vi "VisionExecute.v.vi"(8 "error in (no error)":errorcluster) -> (0 "error out":errorcluster)   [LabVIEW 2025]
uses:
  <vilib>/Rock Robotics/WPI/ThirdParty/JAS_Junk/TrajLib/Trajectory_Library.lvlib
  <vilib>/Rock Robotics/WPI/ThirdParty/PhotonVisionLib/PhotonVisionLib.lvlib
  <vilib>/Rock Robotics/WPI/ThirdParty/PhotonVisionLib/Enum/PhotonPoseStrategy_ENUM.ctl
  VisionGlobal.vi
  <vilib>/Rock Robotics/WPI/ThirdParty/JAS_Junk/TrajLib/TypeDef/TRANSLATION2D.ctl
  <vilib>/Rock Robotics/WPI/ThirdParty/JAS_Junk/TrajLib/TypeDef/ROTATION2D.ctl
  <vilib>/Rock Robotics/WPI/ThirdParty/JAS_Junk/TrajLib/TypeDef/POSE2D.ctl
  VisionNetworkingGlobal.vi
  <vilib>/Rock Robotics/Network Tables/NT Write Number.vi
  <vilib>/Rock Robotics/WPI/ThirdParty/JAS_Junk/TrajLib/VI/AprilTagFieldLayout_New2026AndyMark.vi
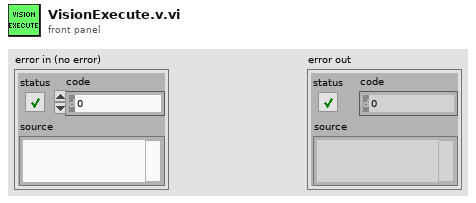
[diagram p1: front panel]
types:
  T1 = typedef "PhotonVisionLib.lvlib/PhotonPoseStrategy_ENUM.ctl" = enum16{"LOWEST_AMBIGUITY", "CLOSEST_TO_CAMERA_HEIGHT", "CLOSEST_TO_REFERENCE_POSE", "CLOSEST_TO_LAST_POSE", "AVERAGE_BEST_TARGETS", "MULTI_TAG_PNP_ON_COPROCESSOR", "MULTI_TAG_PNP_ON_RIO", "PNP_DISTANCE_TRIG_SOLVE", "CONSTRAINED_SOLVEPNP"}
  T2 = typedef "Trajectory_Library.lvlib/TRANSLATION3D.ctl" = cluster{"X":dbl, "Y":dbl, "Z":dbl}
  T3 = typedef "Trajectory_Library.lvlib/ROTATION3D.ctl" = cluster{"Q_quaternion":T4}
  T4 = typedef "Trajectory_Library.lvlib/QUATERNION.ctl" = cluster{"R":dbl, "V":dbl[]}
  T5 = typedef "Trajectory_Library.lvlib/TRANSFORM3D.ctl" = cluster{"TRANSLATION3D":T2, "ROTATION3D":T3, "XF":bool}
  T6 = typedef "PhotonVisionLib.lvlib/PhotonPipelineResultType.ctl" = cluster{"Targets":T7[], "PhotonMultiTargetPNPResult":T9, "PhotonPipelineMetadata":T11}
  T7 = typedef "PhotonVisionLib.lvlib/PhotonTrackedTargetType.ctl" = cluster{"Yaw":dbl, "Pitch":dbl, "Area":dbl, "Skew":dbl, "MinAreaRectCorners":T8[], "BestCameraToTarget":T5, "FiducialId":i32, "AltCameraToTarget":T5, "PoseAmbiguity":dbl, "DetectedCorners":T8[], "ObjDetectId":i32, "ObjDetectConf":sgl}
  T8 = typedef "PhotonVisionLib.lvlib/TargetCornerType.ctl" = cluster{"X":dbl, "Y":dbl}
  T9 = typedef "PhotonVisionLib.lvlib/PhotonMultiTargetPNPResultType.ctl" = cluster{"PhotonPNPResult":T10, "FiducialIDsUsed":i16[]}
  T10 = typedef "PhotonVisionLib.lvlib/PhotonPNPResultType.ctl" = cluster{"IsPresent":bool, "bestReprojErr":dbl, "altReprojErr":dbl, "ambiguity":dbl, "Best":T5, "Alt":T5}
  T11 = typedef "PhotonVisionLib.lvlib/PhotonPipelineMetadataType.ctl" = cluster{"CaptureTimestampMicros":i64, "PublishTimestampMicros":i64, "SequenceID":i64, "TimeSinceLastPong":i64}
  T12 = typedef "Trajectory_Library.lvlib/AprilTagFieldLayout.ctl" = cluster{"AprilTagMap":map{i32, T13}, "FieldLength":dbl, "FieldWidth":dbl, "OriginPosition ":T15, "OriginPose3d":T14}
  T13 = typedef "Trajectory_Library.lvlib/AprilTag.ctl" = cluster{"ID":i32, "POSE3D":T14}
  T14 = typedef "Trajectory_Library.lvlib/POSE3D.ctl" = cluster{"Translation3d":T2, "Rotation3d":T3}
  T15 = typedef "Trajectory_Library.lvlib/AprilTagFieldLayoutOrignPosition_ENUM.ctl" = enum16{"kBlueAllianceWallRightSide,", "kRedAllianceWallRightSide,"}
  T16 = typedef "Trajectory_Library.lvlib/POSE2D.ctl" = cluster{"TRANSLATION":T17, "ROTATION":T18}
  T17 = typedef "Trajectory_Library.lvlib/TRANSLATION2D.ctl" = cluster{"X":dbl, "Y":dbl}
  T18 = typedef "Trajectory_Library.lvlib/ROTATION2D.ctl" = cluster{"VALUE":dbl, "COS":dbl, "SIN":dbl}
  T19 = typedef "PhotonVisionLib.lvlib/PhotonPoseEstimator_Configuration.ctl" = cluster{"Primary Strategy":T1, "Camera":string, "Initial Pose":T14, "HighestAmbiguity":dbl, "RobotToCamera":T5, "FallBack Strategy":T1, "BaseNTName":string}
  T20 = typedef "Trajectory_Library.lvlib/SWERVE_DRIVE_KINEMATICS.ctl" = cluster{"NumModules":i32, "InverseKinematics":T21, "ForwardKinematics":T21, "Modules":T17[], "PrevCoR":T17, "SavedModuleStates":T22[]}
  T21 = typedef "NI_Matrix.lvlib/RealMatrix.ctl" = dbl[][]
  T22 = typedef "Trajectory_Library.lvlib/SWERVE_DRIVE_MODULE_STATE.ctl" = cluster{"Speed":dbl, "Angle":T18}
  T23 = typedef "Trajectory_Library.lvlib/SWERVE_DRIVE_MODULE_POSITION.ctl" = cluster{"Distance":dbl, "Angle":T18, "P":bool}
  T24 = typedef "Trajectory_Library.lvlib/SWERVE_DRIVE_POSE_EST2_CONFIG.ctl" = cluster{"Wheel_Locations M":T17[], "Odom X std dev M":dbl, "Odom Y std dev M":dbl, "Odom Heading std dev Rad":dbl, "Vision X std dev M":dbl, "Vision Y std dev M":dbl, "Vision Heading std dev Rad":dbl}
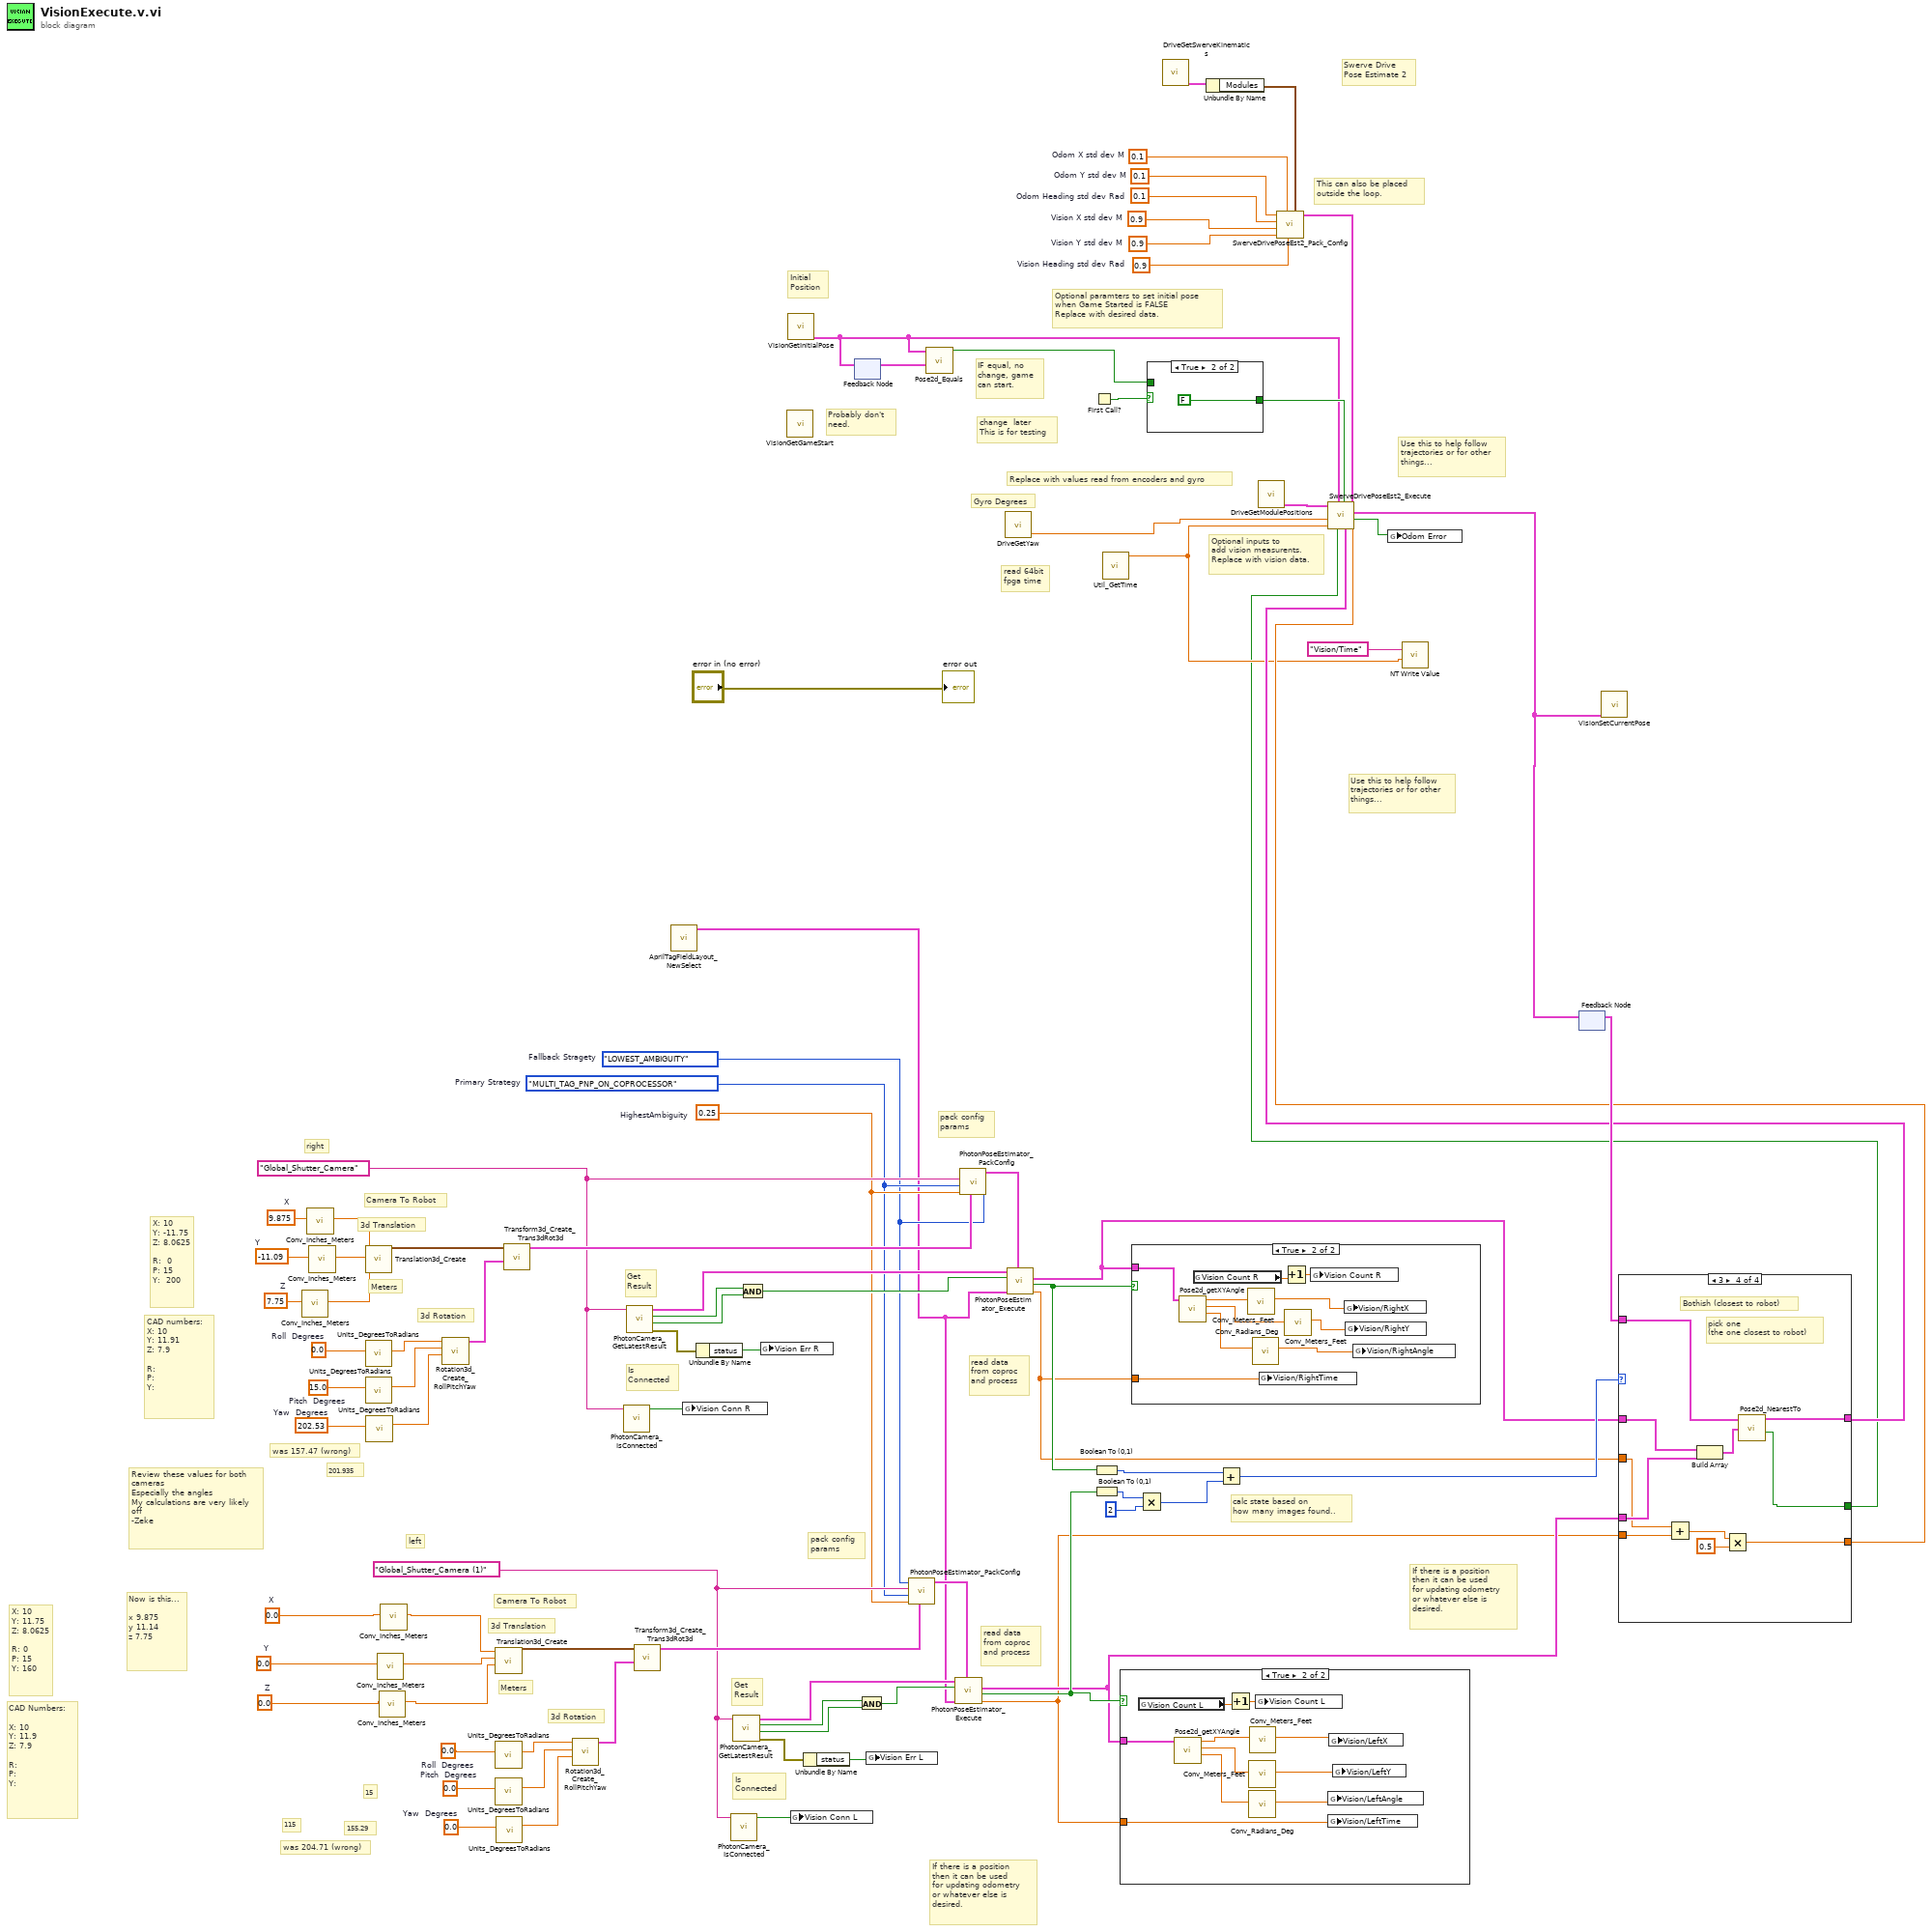
[diagram p0: block diagram]
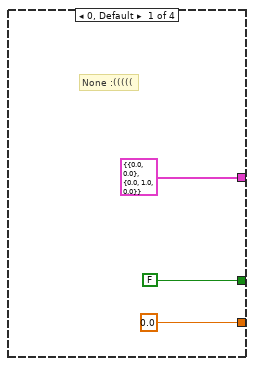
[diagram p3: hidden frame]
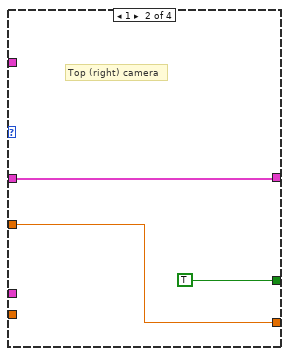
[diagram p4: hidden frame]
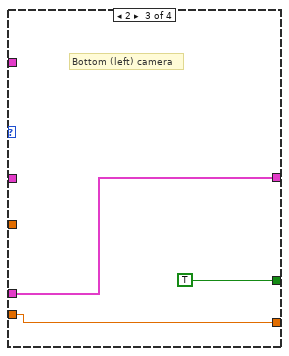
[diagram p5: hidden frame]
diagram:
  w15 = PhotonPoseStrategy_ENUM."LOWEST_AMBIGUITY"  # Fallback Stragety
  w25 = 0.1  # Odom Y std dev M
  w26 = 0.1  # Odom Heading std dev Rad
  w27 = 0.9  # Vision X std dev M
  w28 = 0.9  # Vision Y std dev M
  w29 = 0.1  # Odom X std dev M
  w30 = 0.9  # Vision Heading std dev Rad
  w63 = 0.0  # Roll  Degrees
  w62 = 0.0  # Pitch  Degrees
  w61 = 0.0  # Yaw  Degrees
  w48 = 0.0  # Z
  w52 = 0.0  # X
  w50 = 0.0  # Y
  w57 = "Global_Shutter_Camera (1)" ("CameraName")
  w81 = 0.0  # Roll  Degrees
  w80 = 15.0  # Pitch  Degrees
  w79 = 202.53  # Yaw  Degrees
  w42 = 7.75  # Z
  w46 = 9.875  # X
  w44 = -11.09  # Y
  w40 = 0.25  # HighestAmbiguity
  w39 = PhotonPoseStrategy_ENUM."MULTI_TAG_PNP_ON_COPROCESSOR"  # Primary Strategy
  w75 = "Global_Shutter_Camera" ("CameraName")
  # "calc state based on\nhow many images found.."
  # "read data\nfrom coproc\nand process"
  # "read data\nfrom coproc\nand process"
  # "pack config\nparams"
  # "pack config\nparams"
  # "15"
  # "155.29"
  # "Now is this...\n\nx 9.875\ny 11.14\nz 7.75"
  # "115"
  # "was 157.47 (wrong)"
  # "was 204.71 (wrong)"
  # "CAD Numbers:\n\nX: 10 \nY: 11.9\nZ: 7.9\n\nR:\nP:\nY:"
  # "CAD numbers:\nX: 10\nY: 11.91\nZ: 7.9\n\nR:\nP:\nY:"
  # "X: 10\nY: 11.75\nZ: 8.0625\n\nR: 0\nP: 15\nY: 160"
  # "X: 10 \nY: -11.75\nZ: 8.0625\n\nR:  0\nP: 15\nY:  200"
  # "Probably don't\nneed."
  # "IF equal, no \nchange, game\ncan start."
  # "Initial\nPosition"
  # "201.935"
  # "change  later\nThis is for testing"
  # "Review these values for both cameras\nEspecially the angles\nMy calculations are very likely off\n-Zeke"
  # "Optional inputs to\nadd vision measurents.\nReplace with vision data."
  # "Replace with values read from encoders and gyro"
  # "Optional paramters to set initial pose\nwhen Game Started is FALSE\nReplace with desired data."
  # "read 64bit\nfpga time"
  # "This can also be placed \noutside the loop."
  # "Use this to help follow\ntrajectories or for other\nthings..."
  # "Swerve Drive \nPose Estimate 2"
  # "Use this to help follow\ntrajectories or for other\nthings..."
  # "right"
  # "left"
  # "If there is a position\nthen it can be used\nfor updating odometry\nor whatever else is \ndesired."
  # "Meters"
  # "Camera To Robot"
  # "3d Rotation"
  # "3d Translation"
  # "Is\nConnected"
  # "Get\nResult"
  # "If there is a position\nthen it can be used\nfor updating odometry\nor whatever else is \ndesired."
  # "Meters"
  # "Camera To Robot"
  # "3d Rotation"
  # "3d Translation"
  # "Is\nConnected"
  # "Get\nResult"
  # "Gyro Degrees"
  n1 = call <vilib>:"Conv_Inches_Meters.vi"("INCH"=w42) -> ("Meters"=w41:dbl)  [unwired: 10 in]
  n2 = call <vilib>:"Conv_Inches_Meters.vi"("INCH"=w46) -> ("Meters"=w45:dbl)  [unwired: 10 in]
  n3 = call <vilib>:"Conv_Inches_Meters.vi"("INCH"=w44) -> ("Meters"=w43:dbl)  [unwired: 10 in]
  n4 = call <vilib>:"Translation3d_Create.vi"("Z"=w41, "Y"=w43, "X"=w45) -> ("TRANSLATION3D"=w82:T2)  [unwired: 8 in]
  n5 = call <vilib>:"Units_DegreesToRadians.vi"("Degrees"=w81) -> ("Radians"=w78:dbl)  [unwired: 10 in]
  n6 = call <vilib>:"Units_DegreesToRadians.vi"("Degrees"=w80) -> ("Radians"=w77:dbl)  [unwired: 10 in]
  n7 = call <vilib>:"Units_DegreesToRadians.vi"("Degrees"=w79) -> ("Radians"=w76:dbl)  [unwired: 10 in]
  n8 = call <vilib>:"Conv_Inches_Meters.vi"("INCH"=w50) -> ("Meters"=w49:dbl)  [unwired: 10 in]
  n9 = call <vilib>:"Conv_Inches_Meters.vi"("INCH"=w48) -> ("Meters"=w47:dbl)  [unwired: 10 in]
  n10 = call <vilib>:"Conv_Inches_Meters.vi"("INCH"=w52) -> ("Meters"=w51:dbl)  [unwired: 10 in]
  n11 = call <vilib>:"Rotation3d_Create_RollPitchYaw.vi"("Yaw"=w76, "Pitch"=w77, "Roll"=w78) -> ("Rotation3d"=w83:T3)  [unwired: 8 in]
  n12 = call <vilib>:"Translation3d_Create.vi"("Z"=w47, "Y"=w49, "X"=w51) -> ("TRANSLATION3D"=w64:T2)  [unwired: 8 in]
  n13 = call <vilib>:"Units_DegreesToRadians.vi"("Degrees"=w63) -> ("Radians"=w60:dbl)  [unwired: 10 in]
  n14 = call <vilib>:"Units_DegreesToRadians.vi"("Degrees"=w62) -> ("Radians"=w59:dbl)  [unwired: 10 in]
  n15 = call <vilib>:"Units_DegreesToRadians.vi"("Degrees"=w61) -> ("Radians"=w58:dbl)  [unwired: 10 in]
  n16 = call <vilib>:"Transform3d_Create_Trans3dRot3d.vi"("Rotation3d"=w83, "Translation3d"=w82) -> ("Transform3d"=w84:T5)  [unwired: 9 in]
  n17 = call <vilib>:"Rotation3d_Create_RollPitchYaw.vi"("Yaw"=w58, "Pitch"=w59, "Roll"=w60) -> ("Rotation3d"=w65:T3)  [unwired: 8 in]
  n18 = call <vilib>:"PhotonCamera_IsConnected.vi"("CameraName"=w75) -> ("IsConnected"=w73:bool)  [unwired: 9 in, 1 out]
  n19 = call <vilib>:"PhotonCamera_GetLatestResult.vi"("CameraName"=w75) -> ("error out"=w72:errorcluster, "New Data"=w88:bool, "HasTargets"=w87:bool, "PipelineResult"=w85:T6)  [unwired: 6 in, 1 out]
  n20 = call <vilib>:"Transform3d_Create_Trans3dRot3d.vi"("Rotation3d"=w65, "Translation3d"=w64) -> ("Transform3d"=w66:T5)  [unwired: 9 in]
  n21 = call-poly <vilib>:"AprilTagFieldLayout_NewSelect.vi"() -> ("AprilTagFieldLayout"=w1:T12)  [unwired: 11 in]
  n22 = global write "VisionGlobal.vi" "Vision Conn R"(w73) -> ()
  n23 = Unbundle By Name(w72) -> ("status"=w71:bool)
  n24 = call <vilib>:"PhotonCamera_IsConnected.vi"("CameraName"=w57) -> ("IsConnected"=w55:bool)  [unwired: 9 in, 1 out]
  n25 = call <vilib>:"PhotonCamera_GetLatestResult.vi"("CameraName"=w57) -> ("error out"=w54:errorcluster, "New Data"=w70:bool, "HasTargets"=w69:bool, "PipelineResult"=w67:T6)  [unwired: 6 in, 1 out]
  n26 = And(x=w87, y=w88) -> (x .and. y?=w86:bool)
  n27 = global write "VisionGlobal.vi" "Vision Err R"(w71) -> ()
  n28 = call "VisionGetGameStart.vi"() -> ()  [unwired: 11 in, 1 out]
  n29 = call "VisionGetInitialPose.vi"() -> ("InitialPose"=w5:T16)  [unwired: 10 in]
  n30 = global write "VisionGlobal.vi" "Vision Conn L"(w55) -> ()
  n31 = Unbundle By Name(w54) -> ("status"=w53:bool)
  n32 = feedback-in #1(w5) -> ()
  n33 = feedback #1() -> (w4:T16)  [unwired: 1 in]
  n34 = And(x=w69, y=w70) -> (x .and. y?=w68:bool)
  n35 = global write "VisionGlobal.vi" "Vision Err L"(w53) -> ()
  n36 = call <vilib>:"PhotonPoseEstimator_PackConfig.vi"("FallBack Strategy"=w15, "RobotToCamera"=w66, "HighestAmbiguity"=w40, "PirmaryStrategy"=w39, "Camera"=w57) -> ("PoseEstimator_Configuration"=w56:T19)  [unwired: 6 in]
  n37 = call <vilib>:"Pose2d_Equals.vi"("other POSE"=w4, "in POSE"=w5) -> ("Equals"=w3:bool)  [unwired: 9 in]
  n38 = call <vilib>:"PhotonPoseEstimator_Execute.vi"("Configuration"=w56, "AprilTagFieldLayout"=w1, "PIpeline Has \nNew Results"=w68, "PipelineResult"=w67) -> ("TimeStamp_Seconds"=w10:dbl, "New Pose Found"=w37:bool, "EstimatedPose2d"=w12:T16)  [unwired: 1 in, 4 out]
  n39 = call <vilib>:"PhotonPoseEstimator_PackConfig.vi"("FallBack Strategy"=w15, "RobotToCamera"=w84, "HighestAmbiguity"=w40, "PirmaryStrategy"=w39, "Camera"=w75) -> ("PoseEstimator_Configuration"=w74:T19)  [unwired: 6 in]
  n40 = call "DriveGetYaw.vi"() -> ("Yaw"=w20:dbl)  [unwired: 11 in]
  n41 = call <vilib>:"PhotonPoseEstimator_Execute.vi"("Configuration"=w74, "AprilTagFieldLayout"=w1, "PIpeline Has \nNew Results"=w86, "PipelineResult"=w85) -> ("TimeStamp_Seconds"=w9:dbl, "New Pose Found"=w38:bool, "EstimatedPose2d"=w11:T16)  [unwired: 1 in, 4 out]
  n42 = First Call?() -> (First Call?: T/F=w13:bool)
  n43 = Boolean To (0,1)(Boolean=w38) -> (0, 1=w33:i16)
  n44 = Boolean To (0,1)(Boolean=w37) -> (0, 1=w36:i16)
  n45 = call <vilib>:"Util_GetTime.vi"() -> ("FPGA_Time_Seconds"=w7:dbl)  [unwired: 9 in, 2 out]
  n46 = case shown="True" w37 {
    tunnel: w12 -> [_ w96]
    tunnel: w10 -> [_ w95]
    frame False {
    }
    frame True {
      n47 = global read "VisionGlobal.vi" "Vision Count L"() -> (w97:dbl)
      n48 = call <vilib>:"Pose2d_getXYAngle.vi"("in POSE"=w96) -> ("Angle"=w90:dbl, "Y"=w92:dbl, "X"=w94:dbl)  [unwired: 8 in]
      n49 = Increment(x=w97) -> (x+1=w98:dbl)
      n50 = call <vilib>:"Conv_Meters_Feet.vi"("Meters"=w92) -> ("Feet"=w91:dbl)  [unwired: 10 in]
      n51 = call <vilib>:"Conv_Radians_Deg.vi"("Radians"=w90) -> ("Degrees"=w89:dbl)  [unwired: 10 in]
      n52 = call <vilib>:"Conv_Meters_Feet.vi"("Meters"=w94) -> ("Feet"=w93:dbl)  [unwired: 10 in]
      n53 = global write "VisionGlobal.vi" "Vision Count L"(w98) -> ()
      n54 = global write "VisionNetworkingGlobal.vi" "Vision/LeftAngle"(w89) -> ()
      n55 = global write "VisionNetworkingGlobal.vi" "Vision/LeftTime"(w95) -> ()
      n56 = global write "VisionNetworkingGlobal.vi" "Vision/LeftX"(w93) -> ()
      n57 = global write "VisionNetworkingGlobal.vi" "Vision/LeftY"(w91) -> ()
    }
  }
  n58 = case shown="True" w38 {
    tunnel: w11 -> [_ w106]
    tunnel: w9 -> [_ w105]
    frame False {
    }
    frame True {
      n59 = call <vilib>:"Pose2d_getXYAngle.vi"("in POSE"=w106) -> ("Angle"=w100:dbl, "Y"=w102:dbl, "X"=w104:dbl)  [unwired: 8 in]
      n60 = global read "VisionGlobal.vi" "Vision Count R"() -> (w107:dbl)
      n61 = call <vilib>:"Conv_Meters_Feet.vi"("Meters"=w104) -> ("Feet"=w103:dbl)  [unwired: 10 in]
      n62 = call <vilib>:"Conv_Radians_Deg.vi"("Radians"=w100) -> ("Degrees"=w99:dbl)  [unwired: 10 in]
      n63 = global write "VisionNetworkingGlobal.vi" "Vision/RightTime"(w105) -> ()
      n64 = Increment(x=w107) -> (x+1=w108:dbl)
      n65 = call <vilib>:"Conv_Meters_Feet.vi"("Meters"=w102) -> ("Feet"=w101:dbl)  [unwired: 10 in]
      n66 = global write "VisionGlobal.vi" "Vision Count R"(w108) -> ()
      n67 = global write "VisionNetworkingGlobal.vi" "Vision/RightX"(w103) -> ()
      n68 = global write "VisionNetworkingGlobal.vi" "Vision/RightY"(w101) -> ()
      n69 = global write "VisionNetworkingGlobal.vi" "Vision/RightAngle"(w99) -> ()
    }
  }
  n70 = Multiply(x=w36, y=i16 2) -> (x*y=w34:i16)
  n71 = case shown="True" w13 {
    tunnel: [w109 FALSE] -> w14
    tunnel: w3 -> [w109 _]
    frame False {
    }
    frame True {
    }
  }
  n72 = call "DriveGetSwerveKinematics.vi"() -> ("SWERVE_DRIVE_KINEMATICS"=w17:T20)  [unwired: 11 in]
  n73 = Unbundle By Name(w17) -> ("Modules"=w16:T17[])
  n74 = Add(x=w33, y=w34) -> (x+y=w32:i16)
  n75 = call "DriveGetModulePositions.vi"() -> ("Swerve_Drive_Modual_Positions"=w21:T23[])  [unwired: 11 in]
  n76 = call <vilib>:"SwerveDrivePoseEst2_Pack_Config.vi"("Wheel_Locations M"=w16, "Vision Heading std dev Rad"=w30, "Odom X std dev M"=w29, "Vision Y std dev M"=w28, "Vision X std dev M"=w27, "Odom Heading std dev Rad"=w26, "Odom Y std dev M"=w25) -> ("SwervePoseEst2Config"=w24:T24)  [unwired: 4 in]
  n77 = call-poly <vilib>:"NT Write Value.vi"("value"=w7, "name"="Vision/Time") -> ()  [unwired: 9 in, 1 out]
  n78 = feedback #2() -> (w31:T16)  [unwired: 1 in]
  n79 = case shown="3" w32 {
    tunnel: w11 -> [_ w115 _ w128]
    tunnel: w12 -> [_ _ w118 w127]
    tunnel: w31 -> [_ _ _ w129]
    tunnel: [FALSE ("Found") TRUE ("Found") TRUE ("Found") w125] -> w6
    tunnel: w9 -> [_ w116 _ w124]
    tunnel: w10 -> [_ _ w119 w123]
    tunnel: [T16 {"TRANSLATION"={"X"=0.0, "Y"=0.0}, "ROTATION"={"VALUE"=0.0, "COS"=1.0, "SIN"=0.0}} ("Nearest Pose") w115 w118 w126] -> w19
    tunnel: [0.0 w116 w119 w120] -> w18
    frame 0, Default {
      # "None :((((("
    }
    frame 1 {
      # "Top (right) camera"
    }
    frame 2 {
      # "Bottom (left) camera"
    }
    frame 3 {
      # "pick one \n(the one closest to robot)"
      # "Bothish (closest to robot)"
      n80 = Add(x=w124, y=w123) -> (x+y=w122:dbl)
      n81 = Build Array(w128, w127) -> (w130:T16[])
      n82 = Multiply(x=w122, y=0.5) -> (x*y=w120:dbl)
      n83 = call <vilib>:"Pose2d_NearestTo.vi"("other POSE"=w130, "in POSE"=w129) -> ("Found"=w125:bool, "Nearest Pose"=w126:T16)  [unwired: 8 in]
    }
  }
  n84 = call <vilib>:"SwerveDrivePoseEst2_Execute.vi"("Vision TImeStamp_Seconds"=w18, "SwervePoseEst2Config"=w24, "visionRobotPose"=w19, "Game Started"=w14, "Add Vision Meas"=w6, "InitialPose"=w5, "Pass Through Time"=w7, "Gyro Degrees"=w20, "Module Positions"=w21) -> ("Error"=w22:bool, "Estimated Pose"=w23:T16)  [unwired: 1 in]
  n85 = global write "VisionGlobal.vi" "Odom Error"(w22) -> ()
  n86 = feedback-in #2(w23) -> ()
  n87 = call "VisionSetCurrentPose.vi"("Current Pose"=w23) -> ()  [unwired: 11 in]
  "error out" <- "error in (no error)"
